vi "PH_AWG-510.PC Set Output Settings.vi"(0 "VI in":refnum<vi>, 2 "Wanted Output Settings":T1={"Activate Channel"=FALSE, "VPP (V)"=0.0, "Clock (Hz)"=0.0, "File Name (Device)"="", "#1"=0, "#2"=0, "#3"=0, "#4"=0, "#5"=0, "#6"=0, "#7"=0, "#8"=0, "#9"=0, "#10"=0, "#11"=0, "#12"=0, "#13"=0, "#14"=0, "#15"=0, "#16"=0, "#17"=0, "#18"=0, "#19"=0, "#20"=0, "Offset (V)"=-1.0} {"#20" max=1023 step=1 scale=0.0..1023.0; "#19" max=1023 step=1 scale=0.0..1023.0; "#18" max=1023 step=1 scale=0.0..1023.0; "#17" max=1023 step=1 scale=0.0..1023.0; "#16" max=1023 step=1 scale=0.0..1023.0; "#15" max=1023 step=1 scale=0.0..1023.0; "#14" max=1023 step=1 scale=0.0..1023.0; "#13" max=1023 step=1 scale=0.0..1023.0; "#12" max=1023 step=1 scale=0.0..1023.0; "#11" max=1023 step=1 scale=0.0..1023.0; "#10" max=1023 step=1 scale=0.0..1023.0; "#9" max=1023 step=1 scale=0.0..1023.0; "#8" max=1023 step=1 scale=0.0..1023.0; "#7" max=1023 step=1 scale=0.0..1023.0; "#6" max=1023 step=1 scale=0.0..1023.0; "#5" max=1023 step=1 scale=0.0..1023.0; "#4" max=1023 step=1 scale=0.0..1023.0; "#3" max=1023 step=1 scale=0.0..1023.0; "#2" max=1023 step=1 scale=0.0..1023.0; "#1" max=1023 step=1 scale=0.0..1023.0}, 5 "error in (no error)":errorcluster) -> (14 "VI out":refnum<vi>, 19 "error out":errorcluster)   [LabVIEW 2014, in "PH_AWG-510.lvlib"]
doc: "This VI sets the output settings of the hardware and requests afterwards the current settings to store them on own attributes and to display them at the GUI."
uses:
  PH_AWG-510.lvlib
  PH_AWG-510.Output Settings.ctl
  instr.lib/awg510/Tektronix AWG510 - Driver.lvlib
panel:
  # "Waveform Pattern"
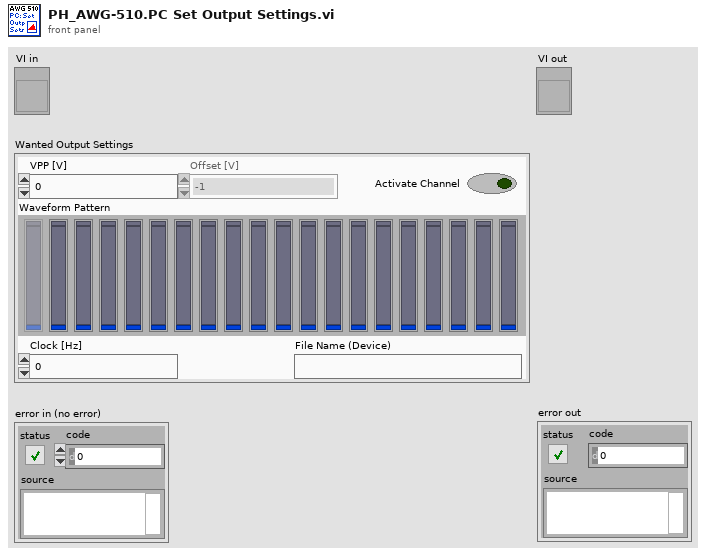
[diagram p1: front panel]
types:
  T1 = typedef "PH_AWG-510.lvlib/PH_AWG-510.Output Settings.ctl" = cluster{"Activate Channel":bool, "VPP (V)":dbl, "Clock (Hz)":dbl, "File Name (Device)":string, "#1":u16, "#2":u16, "#3":u16, "#4":u16, "#5":u16, "#6":u16, "#7":u16, "#8":u16, "#9":u16, "#10":u16, "#11":u16, "#12":u16, "#13":u16, "#14":u16, "#15":u16, "#16":u16, "#17":u16, "#18":u16, "#19":u16, "#20":u16, "Offset (V)":dbl}
  T2 = typedef "PH_AWG-510.lvlib/PH_AWG-510.i attribute.ctl" = cluster{"GUI Refs":cluster{"Delete":refnum<vi>, "Trigger Settings":refnum<vi>, "Start Device":refnum<vi>, "Instrument Information":refnum<vi>, "Lock Frontpanel":refnum<vi>, "Waveform Pattern File":refnum<vi>, "Initialize":refnum<vi>, "Output Settings":refnum<vi>}, "Instrument Information":T3, "Initialized?":bool, "Current Settings":cluster{"Trigger":T4, "Output Settings":T1}, "Wanted Settings":cluster{"Trigger":T4, "Output Settings":T1}, "Device frontpanel locked?":bool, "Default File Path":path}
  T3 = typedef "PH_AWG-510.lvlib/PH_AWG-510.Instrument Information Dataset.ctl" = cluster{"VISA resource name":refnum<visa-resource-name>, "Instrument Firmware Revision":string, "Manufacturer":string, "Model":string, "Serial Number":string, "Error Message":string, "Device Status":enum16{"stopped", "wating for trigger", "running", "Failure"}}
  T4 = typedef "PH_AWG-510.lvlib/PH_AWG-510.Trigger Settings.ctl" = cluster{"Mode":enum16{"Continuous", "Triggered", "Gated", "Enhanced"}, "Level (V)":dbl, "External Source":bool}
  T5 = enum8{"Enabled", "Disabled", "Disabled and Grayed Out"}
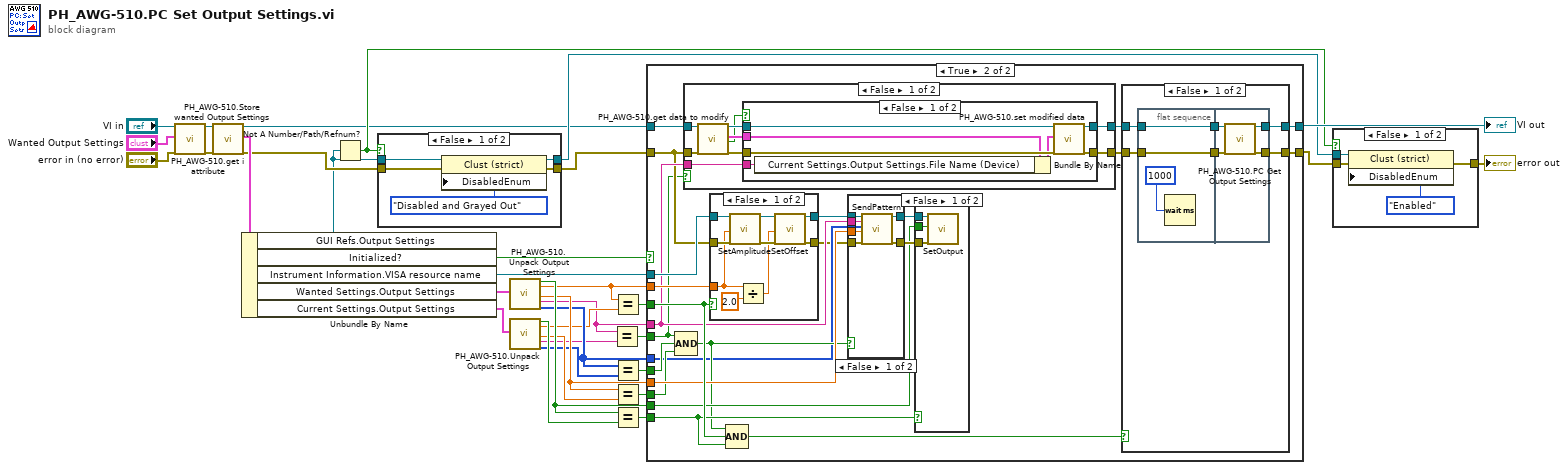
[diagram p0: block diagram]
diagram:
  n1 = call "PH_AWG-510.Store wanted Output Settings.vi"("VI in"="VI in", "Wanted Output Settings"="Wanted Output Settings", "error in (no error)"="error in (no error)") -> ("VI out"=w17:refnum<vi>, "error out"=w16:errorcluster)  [unwired: 15 in]
  n2 = call "PH_AWG-510.get i attribute.vi"("i ref in"=w17, "error in (no error)"=w16) -> ("i ref out"=w15:refnum<vi>, "i attribute"=w34:T2, "error out"=w25:errorcluster)  [unwired: 15 in]
  n3 = Unbundle By Name(w34) -> ("GUI Refs.Output Settings"=w24:refnum<vi>, "Initialized?"=w32:bool, "Instrument Information.VISA resource name"=w33:refnum<visa-resource-name>, "Wanted Settings.Output Settings"=w12:T1, "Current Settings.Output Settings"=w11:T1)
  n4 = Not A Number/Path/Refnum?(number/path/refnum=w24) -> (NaN/Path/Refnum?=w20:bool)
  n5 = case shown="False" w20 {
    tunnel: w25 -> [w39 w41]
    tunnel: [w38 w41] -> w14
    tunnel: w24 -> [w37 w40]
    tunnel: [w35 w40] -> w21
    frame False {
      n6 = property class="Clust (strict)"(reference=w37, error in=w39, "DisabledEnum"=T5."Disabled and Grayed Out" ("Disabled")) -> (reference out=w35:refnum<vi>, error out=w38:errorcluster)
    }
    frame True {
    }
  }
  n7 = call "PH_AWG-510.Unpack Output Settings.vi"("Output Settings"=w12) -> ("Activate Channel"=w10:bool, "VPP [V]"=w4:dbl, "Clock [Hz]"=w7:dbl, "File Name (Device)"=w2:string, "Waveform Pattern"=w6:u16[])  [unwired: 14 in]
  n8 = call "PH_AWG-510.Unpack Output Settings.vi"("Output Settings"=w11) -> ("Activate Channel"=w9:bool, "VPP [V]"=w3:dbl, "Clock [Hz]"=w8:dbl, "File Name (Device)"=w1:string, "Waveform Pattern"=w5:u16[])  [unwired: 14 in]
  n9 = Equal?(x=w2, y=w1) -> (x = y?=w27:bool)
  n10 = Equal?(x=w4, y=w3) -> (x = y?=w31:bool)
  n11 = Equal?(x=w6, y=w5) -> (x = y?=w26:bool)
  n12 = Equal?(x=w7, y=w8) -> (x = y?=w13:bool)
  n13 = Equal?(x=w10, y=w9) -> (x = y?=w28:bool)
  n14 = case shown="True" w32 {
    tunnel: w33 -> [_ w66]
    tunnel: w4 -> [_ w65]
    tunnel: w6 -> [_ w46]
    tunnel: w31 -> [_ w64]
    tunnel: w14 -> [w42 w51]
    tunnel: w15 -> [w43 w55]
    tunnel: [w43 w63] -> w30
    tunnel: [w42 w62] -> w23
    tunnel: w10 -> [_ w57]
    tunnel: w28 -> [_ w56]
    tunnel: w7 -> [_ w60]
    tunnel: w2 -> [_ w54]
    tunnel: w27 -> [_ w47]
    tunnel: w26 -> [_ w48]
    tunnel: w13 -> [_ w49]
    frame False {
    }
    frame True {
      n15 = Compound Arithmetic op=AND(w47, w48, w49) -> (w50:bool)
      n16 = case shown="False" w47 {
        tunnel: w51 -> [w75 w85]
        tunnel: [w73 w85] -> w52
        tunnel: w55 -> [w72 w86]
        tunnel: w54 -> [w69 _]
        tunnel: [w67 w86] -> w53
        frame False {
          n17 = call "PH_AWG-510.get data to modify.vi"("i ref in"=w72, "error in (no error)"=w75) -> ("i ref out"=w71:refnum<vi>, "i attribute"=w70:T2, "timed out"=w68:bool, "error out"=w74:errorcluster)  [unwired: 14 in]
          n18 = case shown="False" w68 {
            tunnel: w74 -> [w82 w84]
            tunnel: [w81 w84] -> w73
            tunnel: w71 -> [w80 w83]
            tunnel: w70 -> [w79 _]
            tunnel: w69 -> [w76 _]
            tunnel: [w77 w83] -> w67
            frame False {
              n19 = Bundle By Name(cluster=w79, "Current Settings.Output Settings.File Name (Device)"=w76) -> (w78:T2)
              n20 = call "PH_AWG-510.set modified data.vi"("i ref in"=w80, "i attribute"=w78, "error in (no error)"=w82) -> ("i ref out"=w77:refnum<vi>, "error out"=w81:errorcluster)  [unwired: 15 in]
            }
            frame True {
            }
          }
        }
        frame True {
        }
      }
      n21 = case shown="False" w64 {
        tunnel: [w117 w123] -> w44
        tunnel: w66 -> [w122 w124]
        tunnel: [w119 w124] -> w45
        tunnel: w51 -> [w121 w123]
        tunnel: w65 -> [w116 _]
        frame False {
          n22 = call "SetAmplitude.vi"("VISA resource name"=w122, "Amplitude (V)"=w116, "error in"=w121) -> ("VISA resource name out"=w120:refnum<visa-resource-name>, "error out"=w118:errorcluster)  [unwired: 15 in]
          n23 = Divide(x=w116, y=2.0) -> (x/y=w114:dbl)
          n24 = call "SetOffset.vi"("VISA resource name"=w120, "Offset (V)"=w114, "error in"=w118) -> ("VISA resource name out"=w119:refnum<visa-resource-name>, "error out"=w117:errorcluster)  [unwired: 15 in]
        }
        frame True {
        }
      }
      n25 = Compound Arithmetic op=AND(w50, w64, w56) -> (w61:bool)
      n26 = case shown="False" w50 {
        tunnel: w44 -> [w110 w112]
        tunnel: w45 -> [w109 w113]
        tunnel: w46 -> [w108 _]
        tunnel: w60 -> [w111 _]
        tunnel: [w107 w112] -> w58
        tunnel: [w106 w113] -> w59
        tunnel: w54 -> [w105 _]
        frame False {
          n27 = call "SendPattern.vi"("VISA resource name"=w109, "File Name (xy.pat)"=w105, "Waveform Pattern"=w108, "Clock (Hz)"=w111, "error in"=w110) -> ("VISA resource name out"=w106:refnum<visa-resource-name>, "error out"=w107:errorcluster)  [unwired: 13 in]
        }
        frame True {
        }
      }
      n28 = case shown="False" w56 {
        tunnel: w59 -> [w89 _]
        tunnel: w58 -> [w88 _]
        tunnel: w57 -> [w87 _]
        frame False {
          n29 = call "SetOutput.vi"("VISA resource name"=w89, "Device on? (true)"=w87, "error in"=w88) -> ()  [unwired: 15 in, 2 out]
        }
        frame True {
        }
      }
      n30 = case shown="False" w61 {
        tunnel: w52 -> [w95 w103]
        tunnel: [w94 w103] -> w62
        tunnel: w53 -> [w93 w104]
        tunnel: [w92 w104] -> w63
        frame False {
          n31 = flat-sequence {
            tunnel: w93 -> [w97]
            tunnel: w95 -> [w98]
            tunnel: [w98] -> w91
            tunnel: [w97] -> w90
            tunnel: [w101] -> w94
            tunnel: [w99] -> w92
            tunnel: w91 -> [w102]
            tunnel: w90 -> [w100]
            frame #0 {
              n32 = Wait (ms)(milliseconds to wait=u32 1000) -> ()  [unwired: 1 out]
            }
            frame #1 {
              n33 = call "PH_AWG-510.PC Get Output Settings.vi"("VI in"=w100, "error in (no error)"=w102) -> ("VI out"=w99:refnum<vi>, "error out"=w101:errorcluster)  [unwired: 16 in]
            }
          }
        }
        frame True {
        }
      }
    }
  }
  "VI out" <- w30
  n34 = case shown="False" w20 {
    tunnel: w23 -> [w128 w129]
    tunnel: [w127 w129] -> w22
    tunnel: w21 -> [w126 _]
    frame False {
      n35 = property class="Clust (strict)"(reference=w126, error in=w128, "DisabledEnum"=T5."Enabled" ("Disabled")) -> (error out=w127:errorcluster)  [unwired: 1 out]
    }
    frame True {
    }
  }
  "error out" <- w22
